vi "BotSpeak.QueueCmd.vi"(4 "String To Send":string, 5 "Bot Settings In":T1) -> (0 "Success?":bool, 1 "String Read":string, 2 "Bot Settings Out":T1)   [LabVIEW 2014]
uses:
  <userlib>/botspeak/VIs/Direct/BotSpeak_Control.ctl
panel:
  out "appended path":path
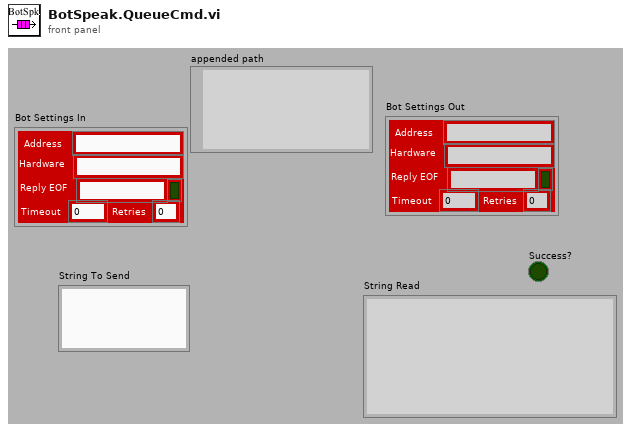
[diagram p1: front panel]
types:
  T1 = typedef "BotSpeak_Control.ctl" = cluster{"Address":string, "Reply EOF":string, "Hardware":string, "Retries":i8, "Timeout":i32, "Open?":bool}
  T2 = enum32{"Bad", "Idle", "Run top level", "Running"}
  T3 = cluster{"Bot Settings In":T1, "String To Send":string, "number: 0 to 1":dbl, string}
  T4 = cluster{"Bot Settings":T1, "String":string, "ID":dbl, "Caller":string}
  T5 = typedef "CommState.ctl" = cluster{"Bot Settings":T1, "Initialized":bool, "Talking":bool}
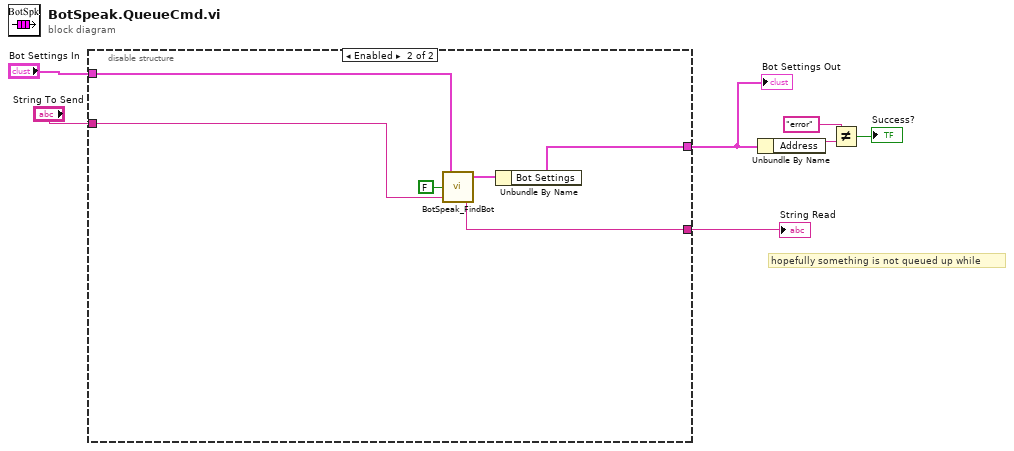
[diagram p0: block diagram]
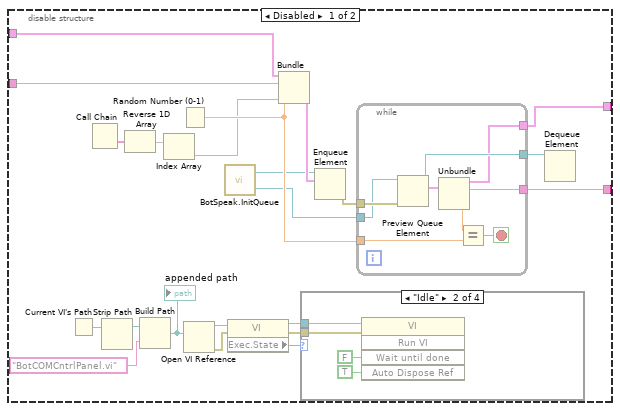
[diagram p2: hidden frame]
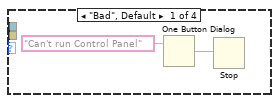
[diagram p3: hidden frame]
diagram:
  # "hopefully something is not queued up while"
  n1 = disable-structure shown="Enabled" {
    disable-tunnel: "String To Send" -> [w29 w49]
    disable-tunnel: [w22 w46] -> w3
    disable-tunnel: [w21 w47] -> w2
    disable-tunnel: "Bot Settings In" -> [w20 w50]
    frame Disabled {
      n2 = Current VI's Path() -> (path=w8:path)
      n3 = Call Chain() -> (call chain=w18:string[])
      n4 = Strip Path(path=w8) -> (stripped path=w9:path)  [unwired: 1 out]
      n5 = Reverse 1D Array(array=w18) -> (reversed array=w17:string[])
      n6 = Build Path(base path=w9, name or relative path="BotCOMCntrlPanel.vi") -> (appended path=w11:path)
      "appended path" <- w11
      n7 = Index Array(array=w17) -> (element=w19:string)  [unwired: 1 in]
      n8 = Random Number (0-1)() -> (number: 0 to 1=w27:dbl)
      n9 = Open VI Reference(vi path=w11) -> (vi reference=w12:refnum<vi>, error out=w13:errorcluster)  [unwired: 5 in]
      n10 = call <userlib>:"BotSpeak.InitQueue.vi"() -> ("ReadQueue"=w25:refnum<queue>, "SendQueue"=w26:refnum<queue>)  [unwired: 2 in]
      n11 = property class="VI"(reference=w12, error in=w13) -> (reference out=w15:refnum<vi>, error out=w16:errorcluster, "Exec.State"=w14:T2)
      n12 = Bundle("Bot Settings In"=w20, "String To Send"=w29, "number: 0 to 1"=w27, w19) -> (w28:T3)  [unwired: 1 in]
      n13 = case shown="\"Idle\"" w14 {
        tunnel: w15 -> [_ w35 _ _]
        tunnel: w16 -> [_ w34 _ _]
        frame "Bad", Default {
          n14 = One Button Dialog(message="Can't run Control Panel") -> (true=w30:bool)  [unwired: 1 in]
          n15 = Stop(stop? (T)=w30) -> ()
        }
        frame "Idle" {
          n16 = invoke class="VI" method="Run VI"(reference=w35, error in=w34, "Wait until done"=FALSE ("Wait Until Done"), "Auto Dispose Ref"=TRUE ("Auto Dispose Reference")) -> ()  [unwired: 1 in, 5 out]
        }
        frame "Run top level" {
        }
        frame "Running" {
        }
      }
      n17 = Enqueue Element(queue=w26, element=w28) -> (error out=w24:errorcluster)  [unwired: 2 in, 2 out]
      n18 = while {
        tunnel: w27 -> [w40]
        tunnel: w25 -> [w41]
        tunnel: w24 -> [w43]
        tunnel: [w38] -> w23
        tunnel: [w37] -> w21
        tunnel: [w36] -> w22
        stop <- w39 stop-if-true
        n19 = Preview Queue Element(queue=w41, error in (no error)=w43) -> (queue out=w38:refnum<queue>, element=w42:T4)  [unwired: 1 in, 2 out]
        n20 = Unbundle(w42) -> ("Bot Settings"=w37:T1, "String"=w36:string, "ID"=w44:dbl)  [unwired: 1 out]
        n21 = Equal?(x=w44, y=w40) -> (x = y?=w39:bool)
      }
      n22 = Dequeue Element(queue=w23) -> ()  [unwired: 2 in, 4 out]
    }
    frame Enabled {
      n23 = call <userlib>:"BotSpeak_FindBot.vi"("String To Send"=w49, "Reset?"=FALSE, "Bot Settings"=w50) -> ("Reply"=w46:string, "Connection"=w48:T5)  [unwired: 1 out]
      n24 = Unbundle By Name(w48) -> ("Bot Settings"=w47:T1)
    }
  }
  "Bot Settings Out" <- w2
  "String Read" <- w3
  n25 = Unbundle By Name(w2) -> ("Address"=w6:string)
  n26 = Not Equal?(x="error", y=w6) -> (x != y?=→"Success?":bool)
